vi "load_OPUS.vi"(0 "fileN":dbl=1.0, 1 "observation":string="ha", 5 "functionpath":path=path "D:/Research/DISCOVER AQ/Data/matlab functions", 7 "spec_path":path=path "D:/Research_CfA/FTS/ha_20150807", 9 "ifg_path":path=path "D:/Research_CfA/FTS/ha_20150807_ifg", 11 "wBound":dbl[][](array[numeric])=[[7765.0, 8005.0], [6180.0, 6260.0], [6297.0, 6382.0], [5880.0, 5996.0], [6007.0, 6145.0]]) -> (3 "spec":dbl[][](array[numeric]), 4 "O2_spec":dbl[][](array[numeric]), 6 "CO2_spec1":dbl[][](array[numeric]), 8 "CO2_spec2":dbl[][](array[numeric]), 10 "CH4_spec1":dbl[][](array[numeric]), 14 "ifg":dbl[](array[numeric]), 15 "CH4_spec2":dbl[][](array[numeric]))   [LabVIEW 2010]
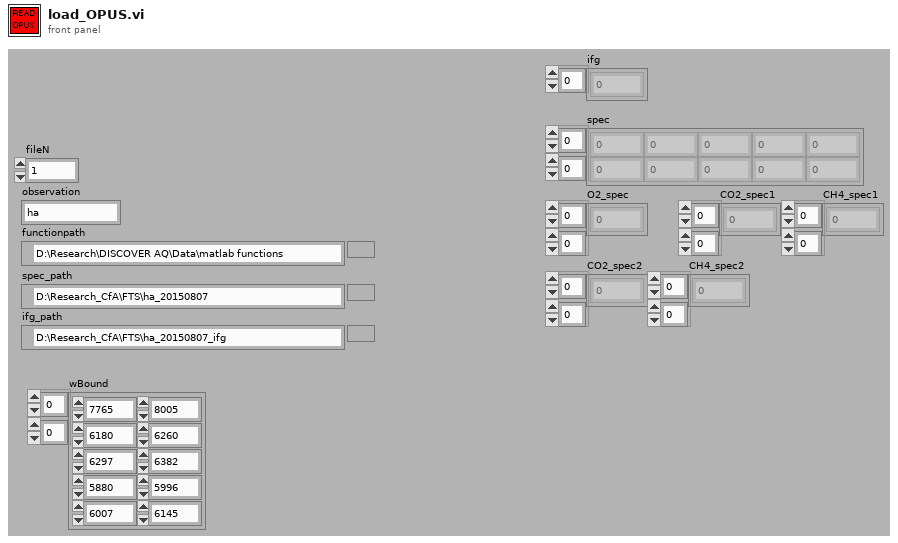
[diagram p1: front panel]
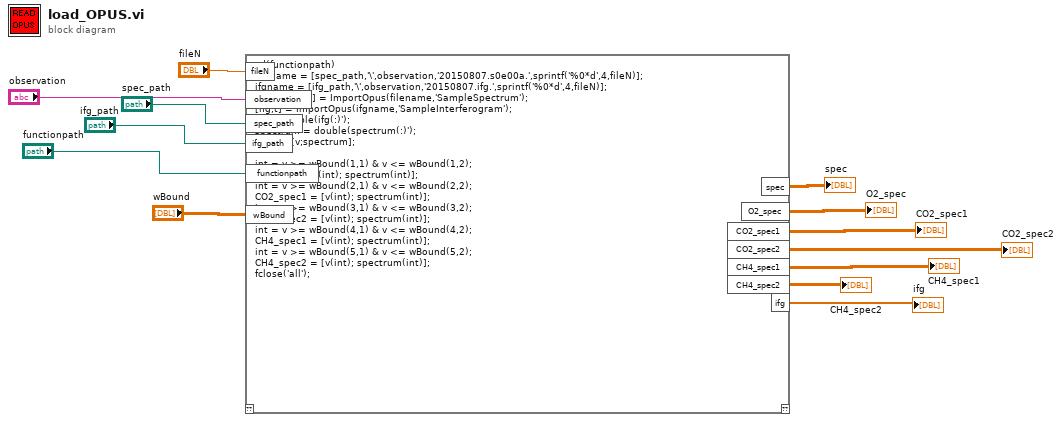
[diagram p0: block diagram]
diagram:
  n1 = script code="cd(functionpath)\nfilename = [spec_path,'\\',observation,'20150807.s0e00a.',sprintf('%0*d',4,fileN)];\nifgname = [ifg_path,'\\',observation,'20150807.ifg.',sprintf('%0*d',4,fileN)];\n[spectrum,v] = ImportOpus(filename,'SampleSpectrum');\n[ifg,t] = ImportOpus(ifgname,'SampleInterferogram');\nifg = double(ifg(:)');\nspectrum = double(spectrum(:)');\nspec = [v;spectrum];\n\nint = v >= wBound(1,1) & v <= wBound(1,2);\nO2_spec = [v(int); spectrum(int)];\nint = v >= wBound(2,1) & v <= wBound(2,2);\nCO2_spec1 = [v(int); spectrum(int)];\nint = v >= wBound(3,1) & v <= wBound(3,2);\nCO2_spec2 = [v(int); spectrum(int)];\nint = v >= wBound(4,1) & v <= wBound(4,2);\nCH4_spec1 = [v(int); spectrum(int)];\nint = v >= wBound(5,1) & v <= wBound(5,2);\nCH4_spec2 = [v(int); spectrum(int)];\nfclose('all');"("observation"="observation", "spec_path"="spec_path", "functionpath"="functionpath", "fileN"="fileN", "ifg_path"="ifg_path", "wBound"="wBound") -> ("O2_spec"=→"O2_spec":dbl[][], "spec"=→"spec":dbl[][], "CO2_spec1"=→"CO2_spec1":dbl[][], "CO2_spec2"=→"CO2_spec2":dbl[][], "CH4_spec1"=→"CH4_spec1":dbl[][], "CH4_spec2"=→"CH4_spec2":dbl[][], "ifg"=→"ifg":dbl[])  [unwired: 1 in, 1 out]
